vi "2 Multiplexers.vi"(8 "6510 Error In":errorcluster, 10 "String":string, 11 "6510 In":refnum<visa-resource-name>) -> (0 "6510 Error Out":errorcluster, 3 "6510 Out":refnum<visa-resource-name>)   [LabVIEW 2019, in "SMU.lvclass"]
uses:
  SMU.lvclass
  <instrlib>/Keithley DMM6500 DAQ6500 Series/Keithley DMM6500 DAQ6500 Series.lvlib
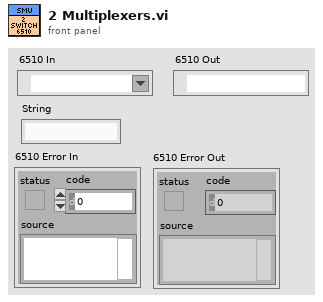
[diagram p1: front panel]
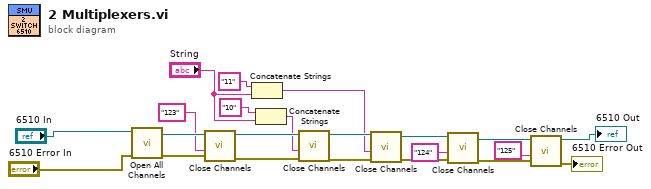
[diagram p0: block diagram]
diagram:
  n1 = call <instrlib>:"Open All Channels.vi"("error in (no error)"="6510 Error In", "VISA resource name"="6510 In") -> ("error out"=w21:errorcluster, "VISA resource name out"=w22:refnum<visa-resource-name>)  [unwired: 8 in]
  n2 = call <instrlib>:"Close Channels.vi"("error in (no error)"=w21, "Channel List(\"\")"="123" ("Channel List(\"\")"), "VISA resource name"=w22) -> ("error out"=w18:errorcluster, "VISA resource name out"=w19:refnum<visa-resource-name>)  [unwired: 7 in]
  n3 = Concatenate Strings("11" ("Channel List(\"\")"), "String") -> (w8:string)
  n4 = Concatenate Strings("10" ("Channel List(\"\")"), "String") -> (w9:string)
  n5 = call <instrlib>:"Close Channels.vi"("error in (no error)"=w18, "Channel List(\"\")"=w9, "VISA resource name"=w19) -> ("error out"=w16:errorcluster, "VISA resource name out"=w17:refnum<visa-resource-name>)  [unwired: 7 in]
  n6 = call <instrlib>:"Close Channels.vi"("error in (no error)"=w16, "Channel List(\"\")"=w8, "VISA resource name"=w17) -> ("error out"=w12:errorcluster, "VISA resource name out"=w13:refnum<visa-resource-name>)  [unwired: 7 in]
  n7 = call <instrlib>:"Close Channels.vi"("error in (no error)"=w12, "Channel List(\"\")"="124" ("Channel List(\"\")"), "VISA resource name"=w13) -> ("error out"=w11:errorcluster, "VISA resource name out"=w14:refnum<visa-resource-name>)  [unwired: 7 in]
  n8 = call <instrlib>:"Close Channels.vi"("error in (no error)"=w11, "Channel List(\"\")"="125" ("Channel List(\"\")"), "VISA resource name"=w14) -> ("error out"=→"6510 Error Out":errorcluster, "VISA resource name out"=→"6510 Out":refnum<visa-resource-name>)  [unwired: 7 in]
